vi "Stop.vi"(8 "error in (no error)":errorcluster, 10 "Message in":refnum<class "StopMessage.lvclass">=refnum, 11 "PockelCell in":refnum<class "PockelCell.lvclass">) -> (0 "error out":errorcluster, 3 "PockelCell out":refnum<class "PockelCell.lvclass">)   [LabVIEW 2012, in "PockelCell.lvclass"]
doc: "This member function is called when the statemachine in the run.vi receives an 'stop' command. It relays the message to all observers of the component.\n\nOverride this member function in your derived class if you need additional stop functionality (but don't forget to call the parent method)."
uses:
  PockelCell.lvclass
  Murmex/LabVIEW/Murmex/StopMessage/StopMessage.lvclass
  <vilib>/Distrio/Murmex/Murmex/Murmex.lvclass
panel:
  # "This method is called when the STOP\ntrigger is sent. \n\nOverride this method when your component needs to\nrespond to this trigger. \n\nCall parent for proper implementation"
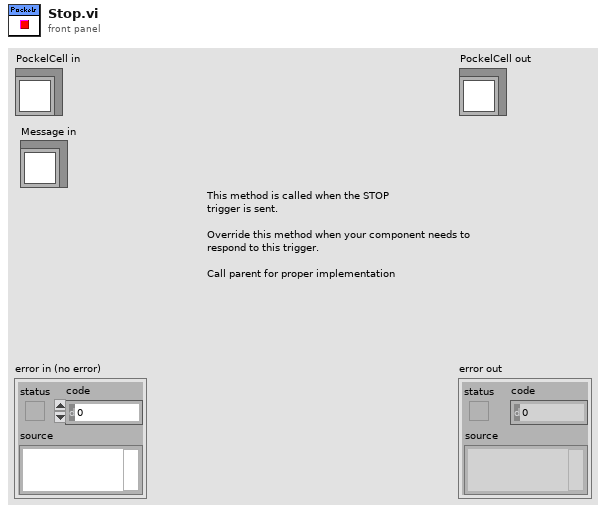
[diagram p1: front panel]
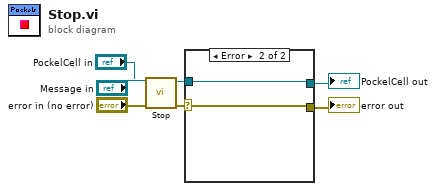
[diagram p0: block diagram]
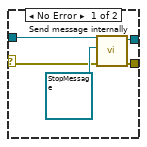
[diagram p2: hidden frame]
diagram:
  n1 = call-parent "Stop.vi"("error in (no error)"="error in (no error)", "Message in"="Message in", "Murmex in"="PockelCell in") -> ("error out"=w4:errorcluster, "Murmex out"=w2:refnum<class "PockelCell.lvclass">)  [unwired: 7 in]
  n2 = case shown="Error" w4 {
    selector: w4 -> [w11 w14]
    tunnel: [w10 w14] -> w3
    tunnel: w2 -> [w9 w13]
    tunnel: [w8 w13] -> w1
    frame No Error {
      n3 = call "Send message internally.vi"("error in (no error)"=w11, "Message"=refnum<class "StopMessage.lvclass"> refnum ("StopMessage.lvclass"), "Murmex in"=w9) -> ("error out"=w10:errorcluster, "Murmex out"=w8:refnum<class "PockelCell.lvclass">)  [unwired: 7 in]
    }
    frame Error {
    }
  }
  "error out" <- w3
  "PockelCell out" <- w1
